vi "close sys config device.vi"(8 "error in":errorcluster, 11 "Controller in":refnum<class "Controller.lvclass">) -> (0 "error out":errorcluster)   [LabVIEW 2016, in "SMI.lvlib" / "SysCfg Device.lvclass"]
uses:
  SysCfg Device.lvclass
  Controller/Controller.lvclass
  C:/GitHub/SystemManagementAndInformation/source/classes/SysCfg Device/SysCfg Device.lvclass
  SysCfg Device.lvclass/SysCfg Device.ctl
  Controller/Controller.lvclass/Controller.ctl
  <vilib>/nisyscfg/Close (System).vi
  <vilib>/nisyscfg/Close (Hardware).vi
  <vilib>/nisyscfg/nisyscfg.lvlib
panel:
  out "Controller out":refnum<class "Controller.lvclass">
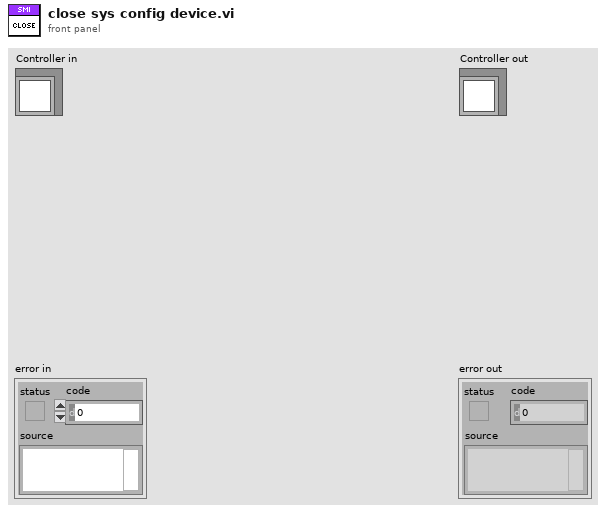
[diagram p1: front panel]
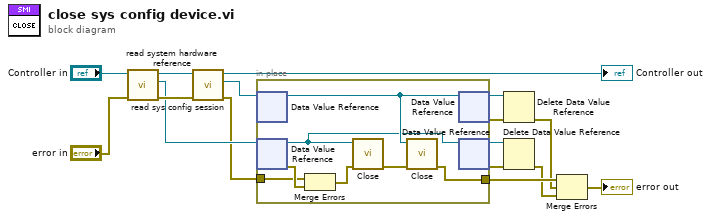
[diagram p0: block diagram]
diagram:
  n1 = call "read system hardware reference.vi"("error in"="error in", "Controller in"="Controller in") -> ("error out"=w13:errorcluster, "system hardware ref"=w11:refnum<data-value>, "Controller out"=w15:refnum<class "Controller.lvclass">)  [unwired: 7 in]
  n2 = call "read sys config session.vi"("error in"=w13, "SysCfg Device in"=w15) -> ("error out"=w10:errorcluster, "sys config session"=w12:refnum<data-value>, "SysCfg Device out"=→"Controller out":refnum<class "Controller.lvclass">)  [unwired: 7 in]
  n3 = in-place {
    in-place-border: w10 -> [w22]
    in-place-border: [w19] -> w9
    n4 = in-place-dvr #1(w12) -> (w18:refnum<k21>)  [unwired: 1 out]
    n5 = in-place-dvr #2(w11) -> (w17:refnum<k20>, w23:errorcluster)
    n6 = Merge Errors(w22, w23) -> (w21:errorcluster)
    n7 = call-poly <vilib>:"Close.vi"("error in (no error)"=w21, "Resource in"=w17) -> ("error out"=w20:errorcluster)  [unwired: 9 in]
    n8 = call-poly <vilib>:"Close.vi"("error in (no error)"=w20, "Session in"=w18) -> ("error out"=w19:errorcluster)  [unwired: 9 in]
    n9 = in-place-dvr #1(w18) -> (w7:refnum<data-value>, w6:errorcluster)
    n10 = in-place-dvr #2(w17) -> (w5:refnum<data-value>, w4:errorcluster)
  }
  n11 = Delete Data Value Reference(data value reference=w7, error in=w6) -> (error out=w3:errorcluster)  [unwired: 1 out]
  n12 = Delete Data Value Reference(data value reference=w5, error in=w4) -> (error out=w2:errorcluster)  [unwired: 1 out]
  n13 = Merge Errors(w9, w3, w2) -> (→"error out":errorcluster)
